vi "Surface_modularity.vi"(2 "Data in":string[][](array[string]), 3 "Channel names":string[](array[string])) -> (0 "Data out":string[][](array[string]))   [LabVIEW 2010]
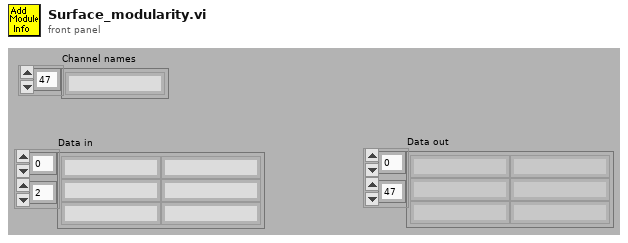
[diagram p1: front panel]
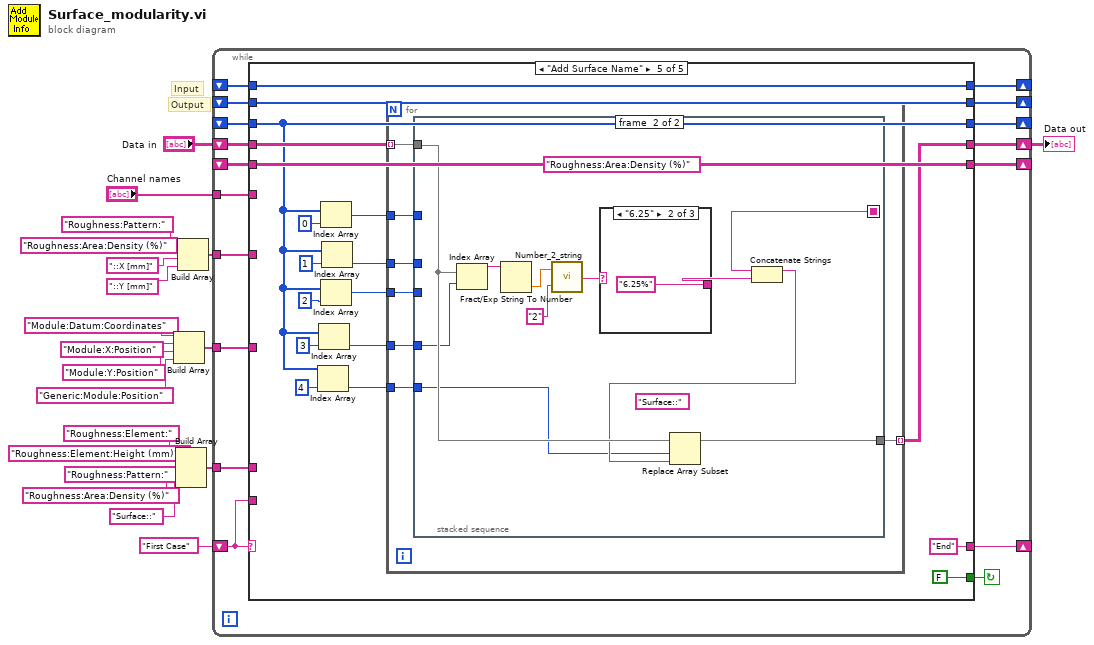
[diagram p0: block diagram]
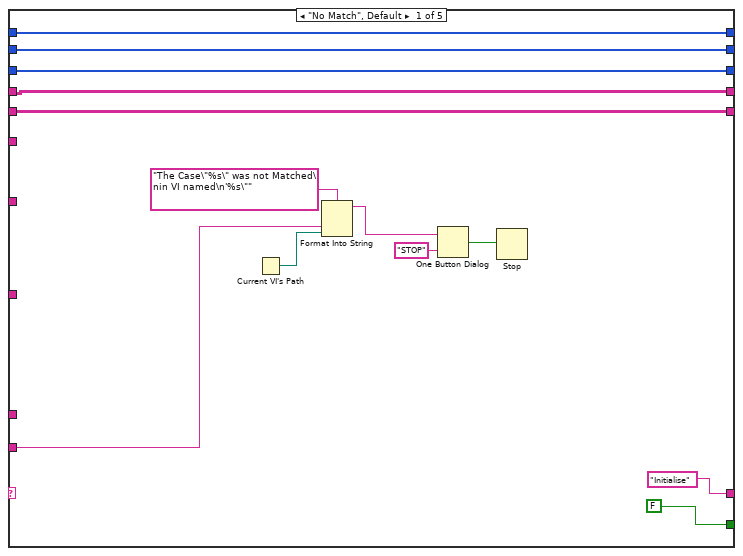
[diagram p2: hidden frame]
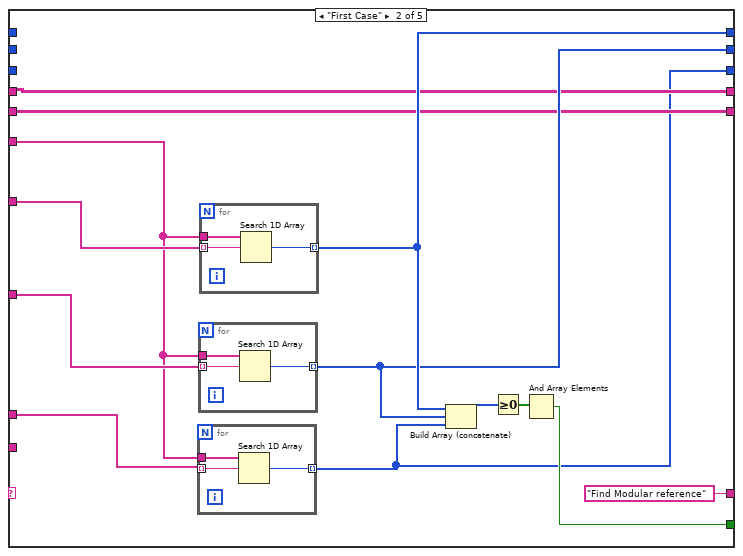
[diagram p3: hidden frame]
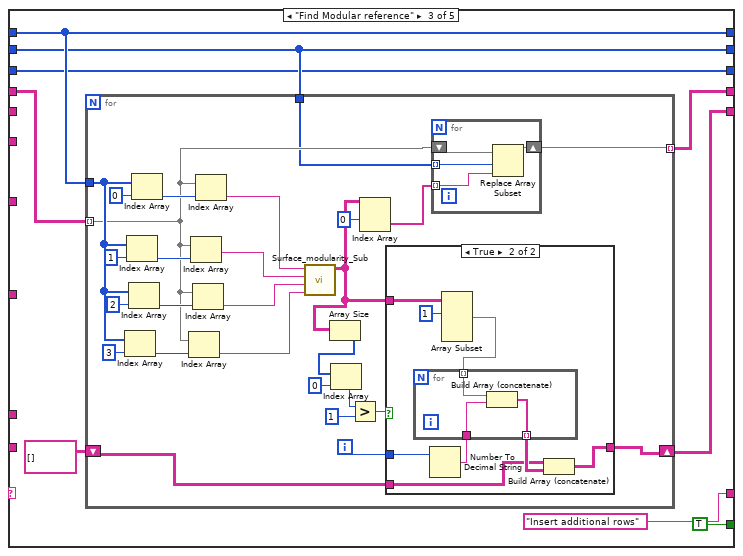
[diagram p4: hidden frame]
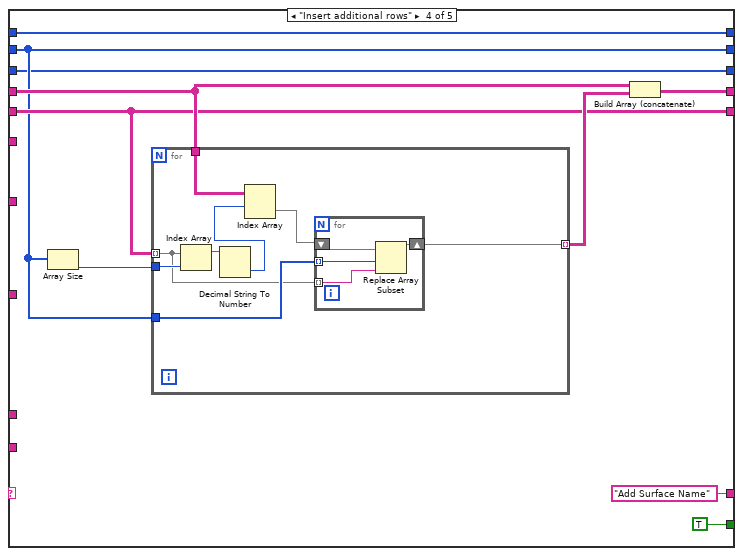
[diagram p6: hidden frame]
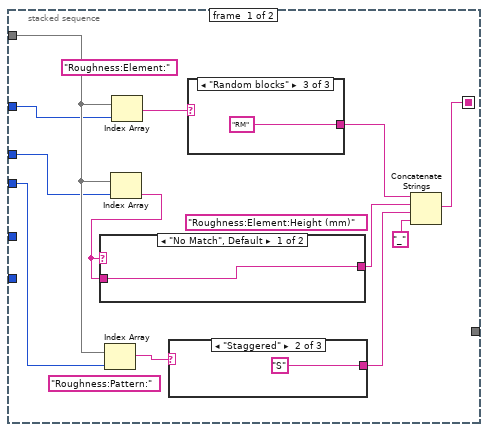
[diagram p7: hidden frame]
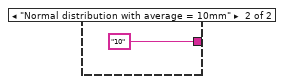
[diagram p8: hidden frame]
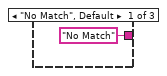
[diagram p9: hidden frame]
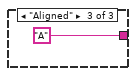
[diagram p10: hidden frame]
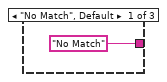
[diagram p11: hidden frame]
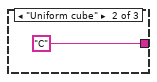
[diagram p12: hidden frame]
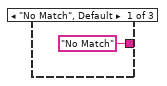
[diagram p13: hidden frame]
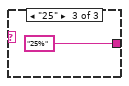
[diagram p14: hidden frame]
diagram:
  # "Output"
  # "Input"
  n1 = Build Array("Module:Datum:Coordinates", "Module:X:Position", "Module:Y:Position", "Generic:Module:Position") -> (w9:string[])
  n2 = Build Array("Roughness:Element:", "Roughness:Element:Height (mm)", "Roughness:Pattern:", "Roughness:Area:Density (%)", "Surface::") -> (w1:string[])
  n3 = Build Array("Roughness:Pattern:", "Roughness:Area:Density (%)", "::X [mm]", "::Y [mm]") -> (w10:string[])
  n4 = while {
    shift-left: "First Case" -> [w35]
    shift-right: [w36] -> _
    shift-right: [w32] -> _
    shift-left: _ -> [w29]
    shift-right: [w30] -> _
    shift-left: _ -> [w28]
    tunnel: "Channel names" -> [w34]
    tunnel: w10 -> [w33]
    tunnel: w9 -> [w31]
    shift-right: [w26] -> w7
    shift-left: "Data in" -> [w27]
    shift-right: [w25] -> _
    shift-left: _ -> [w24]
    tunnel: w1 -> [w23]
    shift-right: [w22] -> _
    shift-left: _ -> [w21]
    stop <- w37 continue-if-true
    n5 = case shown="\"Add Surface Name\"" w35 {
      tunnel: [FALSE w55 TRUE TRUE FALSE] -> w37
      tunnel: ["Initialise" "Find Modular reference" "Insert additional rows" "Add Surface Name" "End"] -> w36
      tunnel: w35 -> [w45 _ _ _ _]
      tunnel: w34 -> [_ w53 _ _ _]
      tunnel: w33 -> [_ w62 _ _ _]
      tunnel: [w42 w60 w80 w134 w164] -> w32
      tunnel: w31 -> [_ w61 _ _ _]
      tunnel: [w41 w59 w79 w128 w160] -> w30
      tunnel: w29 -> [w42 _ w80 w134 w164]
      tunnel: w28 -> [w41 _ w79 w128 w160]
      tunnel: w27 -> [w40 w56 w81 w131 w159]
      tunnel: [w40 w56 w76 w130 w158] -> w26
      tunnel: [w39 w54 w74 w129 w161] -> w25
      tunnel: w24 -> [w39 w54 _ w129 w161]
      tunnel: w23 -> [_ w52 _ _ _]
      tunnel: [w38 w51 w73 w125 w147] -> w22
      tunnel: w21 -> [w38 _ w73 w125 w147]
      frame "No Match", Default {
        n6 = Current VI's Path() -> (path=w44:path)
        n7 = Format Into String(format string="The Case\"%s\" was not Matched\nin VI named\n'%s\"" ("Format String"), w45, w44) -> (resulting string=w48:string)  [unwired: 2 in, 1 out]
        n8 = One Button Dialog(message=w48, button name ("OK")="STOP") -> (true=w46:bool)
        n9 = Stop(stop? (T)=w46) -> ()
      }
      frame "First Case" {
        n10 = for {
          tunnel: w53 -> [w66]
          tunnel: w52 -> [w65] mode=indexing
          tunnel: [w64] -> w51 mode=indexing
          n11 = Search 1D Array(1D array=w66, element=w65) -> (index of element=w64:i32)  [unwired: 1 out]
        }
        n12 = for {
          tunnel: w53 -> [w69]
          tunnel: w61 -> [w68] mode=indexing
          tunnel: [w67] -> w59 mode=indexing
          n13 = Search 1D Array(1D array=w69, element=w68) -> (index of element=w67:i32)  [unwired: 1 out]
        }
        n14 = for {
          tunnel: w53 -> [w72]
          tunnel: w62 -> [w71] mode=indexing
          tunnel: [w70] -> w60 mode=indexing
          n15 = Search 1D Array(1D array=w72, element=w71) -> (index of element=w70:i32)  [unwired: 1 out]
        }
        n16 = Build Array (concatenate)(w60, w59, w51) -> (w58:i32[])
        n17 = Greater Or Equal To 0?(x=w58) -> (x >= 0?=w57:bool[])
        n18 = And Array Elements(Boolean array=w57) -> (logical AND=w55:bool)
      }
      frame "Find Modular reference" {
        n19 = for {
          tunnel: w80 -> [w100]
          tunnel: w81 -> [w99] mode=indexing
          tunnel: w79 -> [w96]
          tunnel: [w93] -> w76 mode=indexing
          shift-right: [w84] -> w74
          shift-left: string[][] [] -> [w85]
          i -> [w86]
          n20 = Index Array(array=w100, index=3) -> (element=w102:i32)
          n21 = Index Array(array=w100, index=1) -> (element=w106:i32)
          n22 = Index Array(array=w100, index=2) -> (element=w103:i32)
          n23 = Index Array(array=w100, index=0) -> (element=w107:i32)
          n24 = Index Array(array=w99, index=w102) -> (element=w82:string)
          n25 = Index Array(array=w99, index=w106) -> (element=w97:string)
          n26 = Index Array(array=w99, index=w103) -> (element=w83:string)
          n27 = Index Array(array=w99, index=w107) -> (element=w98:string)
          n28 = call "Surface_modularity_Sub.vi"("Y Position"=w82, "X Position"=w83, "Roughness Density"=w97, "Roughness Pattern"=w98) -> ("Output values"=w87:string[][])  [unwired: 1 in, 3 out]
          n29 = Array Size(array=w87) -> (size(s)=w92:i32[])
          n30 = Index Array(array=w92, index=0) -> (element=w90:i32)
          n31 = Greater?(x=w90, y=1) -> (0:w88:bool)
          n32 = Index Array(array=w87, index (row)=0) -> (element=w94:string[])  [unwired: 1 in]
          n33 = case shown="True" w88 {
            tunnel: w87 -> [_ w117]
            tunnel: w86 -> [_ w114]
            tunnel: w85 -> [w109 w110]
            tunnel: [w109 w111] -> w84
            frame False {
            }
            frame True {
              n34 = Number To Decimal String(number=w114) -> (decimal integer string=w113:string)  [unwired: 1 out]
              n35 = Array Subset(array=w117, index (row)=1 ("index")) -> (w115:string[][])  [unwired: 3 in]
              n36 = for {
                tunnel: w115 -> [w120] mode=indexing
                tunnel: w113 -> [w119]
                tunnel: [w118] -> w112 mode=indexing
                n37 = Build Array (concatenate)(w120, w119) -> (w118:string[])
              }
              n38 = Build Array (concatenate)(w110, w112) -> (w111:string[][])
            }
          }
          n39 = for {
            shift-right: [w123] -> w93
            shift-left: w99 -> [w124]
            tunnel: w96 -> [w122] mode=indexing
            tunnel: w94 -> [w121] mode=indexing
            n40 = Replace Array Subset(array=w124, new element=w121, index=w122) -> (w123:string[])
          }
        }
      }
      frame "Insert additional rows" {
        n41 = Array Size(array=w128) -> (size(s)=w133:i32)
        n42 = for {
          tunnel: w133 -> [w142]
          tunnel: w129 -> [w136] mode=indexing
          tunnel: w131 -> [w135]
          tunnel: [w138] -> w132 mode=indexing
          tunnel: w128 -> [w137]
          n43 = Index Array(array=w136, index=w142) -> (element=w141:string)
          n44 = Decimal String To Number(string=w141) -> (number=w140:i32)  [unwired: 3 out]
          n45 = Index Array(array=w135, index (row)=w140) -> (element=w139:string[])  [unwired: 1 in]
          n46 = for {
            shift-right: [w145] -> w138
            shift-left: w139 -> [w146]
            tunnel: w137 -> [w144] mode=indexing
            tunnel: w136 -> [w143] mode=indexing
            n47 = Replace Array Subset(array=w146, new element=w143, index=w144) -> (w145:string[])
          }
        }
        n48 = Build Array (concatenate)(w131, w132) -> (w130:string[][])
      }
      frame "Add Surface Name" {
        n49 = Index Array(array=w147, index=4) -> (element=w148:i32)
        n50 = Index Array(array=w147, index=3) -> (element=w149:i32)
        n51 = Index Array(array=w147, index=0) -> (element=w152:i32)
        n52 = Index Array(array=w147, index=2) -> (element=w150:i32)
        n53 = Index Array(array=w147, index=1) -> (element=w151:i32)
        n54 = for {
          tunnel: w159 -> [w171] mode=indexing
          tunnel: [w170] -> w158 mode=indexing
          tunnel: w152 -> [w169]
          tunnel: w151 -> [w168]
          tunnel: w150 -> [w167]
          tunnel: w149 -> [w166]
          tunnel: w148 -> [w165]
          n55 = stacked-sequence {
            seq-local: [w177 _] -> [_ w202]
            tunnel: w171 -> [w180 w200]
            tunnel: [_ w198] -> w170
            tunnel: w169 -> [w176 _]
            tunnel: w168 -> [w175 _]
            tunnel: w167 -> [w174 _]
            tunnel: w166 -> [_ w197]
            tunnel: w165 -> [_ w196]
            frame #0 {
              (unwired) "Roughness:Element:Height (mm)"
              (unwired) "Roughness:Pattern:"
              (unwired) "Roughness:Element:"
              n56 = Index Array(array=w180, index=w174) -> (element=w181:string)
              n57 = Index Array(array=w180, index=w175) -> (element=w172:string)
              n58 = case shown="\"No Match\", Default" w172 {
                tunnel: [w184 "10"] -> w173
                tunnel: w172 -> [w184 _]
                frame "No Match", Default {
                }
                frame "Normal distribution with average = 10mm" {
                }
              }
              n59 = Index Array(array=w180, index=w176) -> (element=w179:string)
              n60 = case shown="\"Staggered\"" w181 {
                tunnel: ["No Match" "S" "A"] -> w182
                frame "No Match", Default {
                }
                frame "Staggered" {
                }
                frame "Aligned" {
                }
              }
              n61 = case shown="\"Random blocks\"" w179 {
                tunnel: ["No Match" "C" "RM"] -> w183
                frame "No Match", Default {
                }
                frame "Uniform cube" {
                }
                frame "Random blocks" {
                }
              }
              n62 = Concatenate Strings(w183, w173, w182, "_") -> (w177:string)
            }
            frame #1 {
              (unwired) "Surface::"
              (unwired) "Roughness:Area:Density (%)"
              n63 = Index Array(array=w200, index=w197) -> (element=w195:string)
              n64 = Fract/Exp String To Number(string=w195) -> (number=w194:dbl)  [unwired: 4 out]
              n65 = call "Number_2_string.vi"("precision"="2", "number"=w194) -> ("String"=w193:string)
              n66 = case shown="\"6.25\"" w193 {
                tunnel: ["No Match" "6.25%" "25%"] -> w201
                frame "No Match", Default {
                }
                frame "6.25" {
                }
                frame "25" {
                }
              }
              n67 = Concatenate Strings(w202, w201) -> (w199:string)
              n68 = Replace Array Subset(array=w200, new element=w199, index=w196) -> (w198:string[])
            }
          }
        }
      }
    }
  }
  "Data out" <- w7
